vi "TimerDemo_2010.vi"   [LabVIEW 2010]
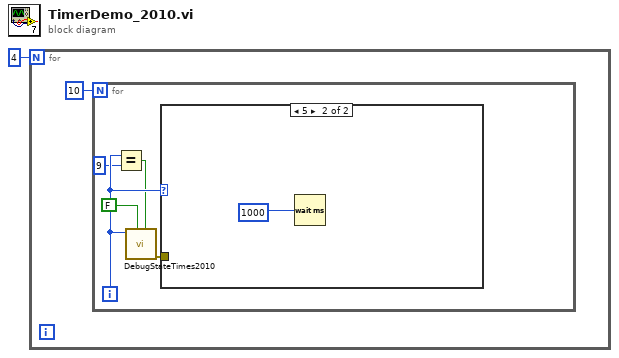
[diagram p0: block diagram]
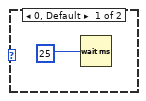
[diagram p2: hidden frame]
diagram:
  n1 = for {
    N: 4 -> [_]
    n2 = for {
      N: 10 -> [_]
      i -> [w6]
      n3 = Equal?(x=w6, y=9) -> (x = y?=w4:bool)
      n4 = call "DebugStateTimes2010.vi"("ShowGUI"=w4, "reset"=FALSE, "iteration"=w6) -> ("error out"=w3:errorcluster)  [unwired: 7 in, 1 out]
      n5 = case shown="5" w6 {
        tunnel: w3 -> [_ _]
        frame 0, Default {
          n6 = Wait (ms)(milliseconds to wait=25 ("y")) -> ()  [unwired: 1 out]
        }
        frame 5 {
          n7 = Wait (ms)(milliseconds to wait=1000 ("y")) -> ()  [unwired: 1 out]
        }
      }
    }
  }
